vi "Launcher.vi"   [LabVIEW 2019]
uses:
  Server/Server/Server.lvclass
  C:/Program Files (x86)/National Instruments/LabVIEW 2019/vi.lib/ActorFramework/Actor/Actor.lvclass
  <vilib>/ActorFramework/Actor/Actor.lvclass
panel:
  # "Launcher"
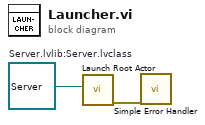
[diagram p0: block diagram]
diagram:
  w1 = refnum<class "Server.lvclass"> refnum  # Server.lvlib:Server.lvclass
  n1 = call <vilib>:"Launch Root Actor.vi"("Actor"=w1) -> ("error out"=w2:errorcluster)  [unwired: 9 in, 1 out]
  n2 = call <vilib>:"Simple Error Handler.vi"("error in (no error)"=w2) -> ()  [unwired: 4 in, 5 out]
